vi "RunFFT.vi"(2 "working directory":path=path "", 3 "spctdata":string, 4 "timedata":string) -> (0 "standard error":string, 1 "standard output":string)   [LabVIEW 2020]
doc: "This VI will compute the FFT of the data located in the file named spctdata, timedata is needed to determine the delta between measurements. Computed FFT data is written to a file named spctdata_Abs_FFT_data and frequency space data is written to the file scpct_data_Frq_data\n\nYou must tell LabVIEW the location of the executable\n\nYou must tell LabVIEW what directory you are working in\n\nWait Until Completion is always set to true\n\nR. Sheehan 7 - 12 - 2018"
panel:
  out "Cmd":string="C:\\Users\\Robert\\Programming\\LabVIEW\\FFT_cmdl\\FFTCalc"
  out "return code":i32
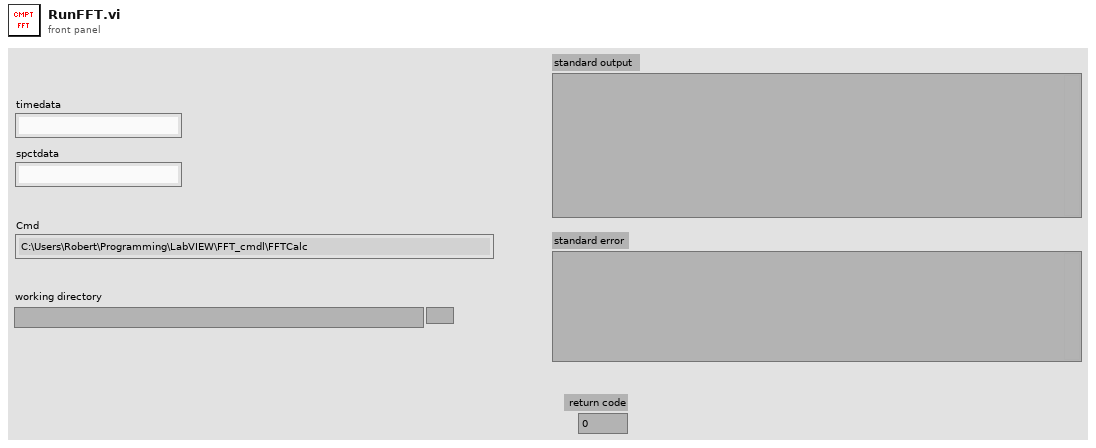
[diagram p1: front panel]
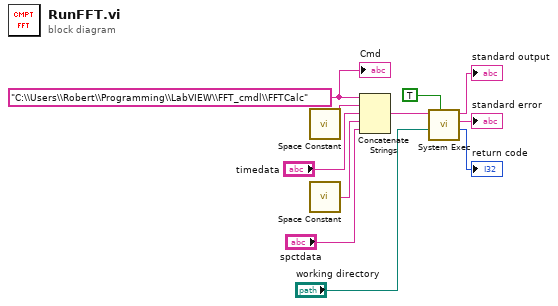
[diagram p0: block diagram]
diagram:
  w7 = "C:\\Users\\Robert\\Programming\\LabVIEW\\FFT_cmdl\\FFTCalc" ("string")
  n1 = call <vilib>:"Space Constant.vi"() -> ("String"=w6:string)
  n2 = call <vilib>:"Space Constant.vi"() -> ("String"=w4:string)
  n3 = Concatenate Strings(w7, w6, "timedata", w4, "spctdata") -> (w2:string)
  n4 = call <vilib>:"System Exec.vi"("wait until completion? (T)"=TRUE, "working directory"="working directory", "command line"=w2) -> ("return code"=→"return code":i32, "standard error"=→"standard error":string, "standard output"=→"standard output":string)  [unwired: 5 in, 1 out]
  "Cmd" <- w7
